vi "Aula03_25022026_Medidor.vi"() -> (0 "Corrente fase C":dynamicdata(graph), 1 "Corrente Fase B":dynamicdata(graph), 2 "Tensão Fase B":dynamicdata(graph), 4 "Tensão Fase C":dynamicdata(graph), 5 "Corrente Fase A":dynamicdata(graph), 6 "Tensão fase A":dynamicdata(graph))   [LabVIEW 2020]
panel:
  out "Fase C":string[][](table)
  out "Fase B":string[][](table)
  out "Fase A":string[][](table)
  out "Fase A":string[][](table)
  out "Table":string[][](table)
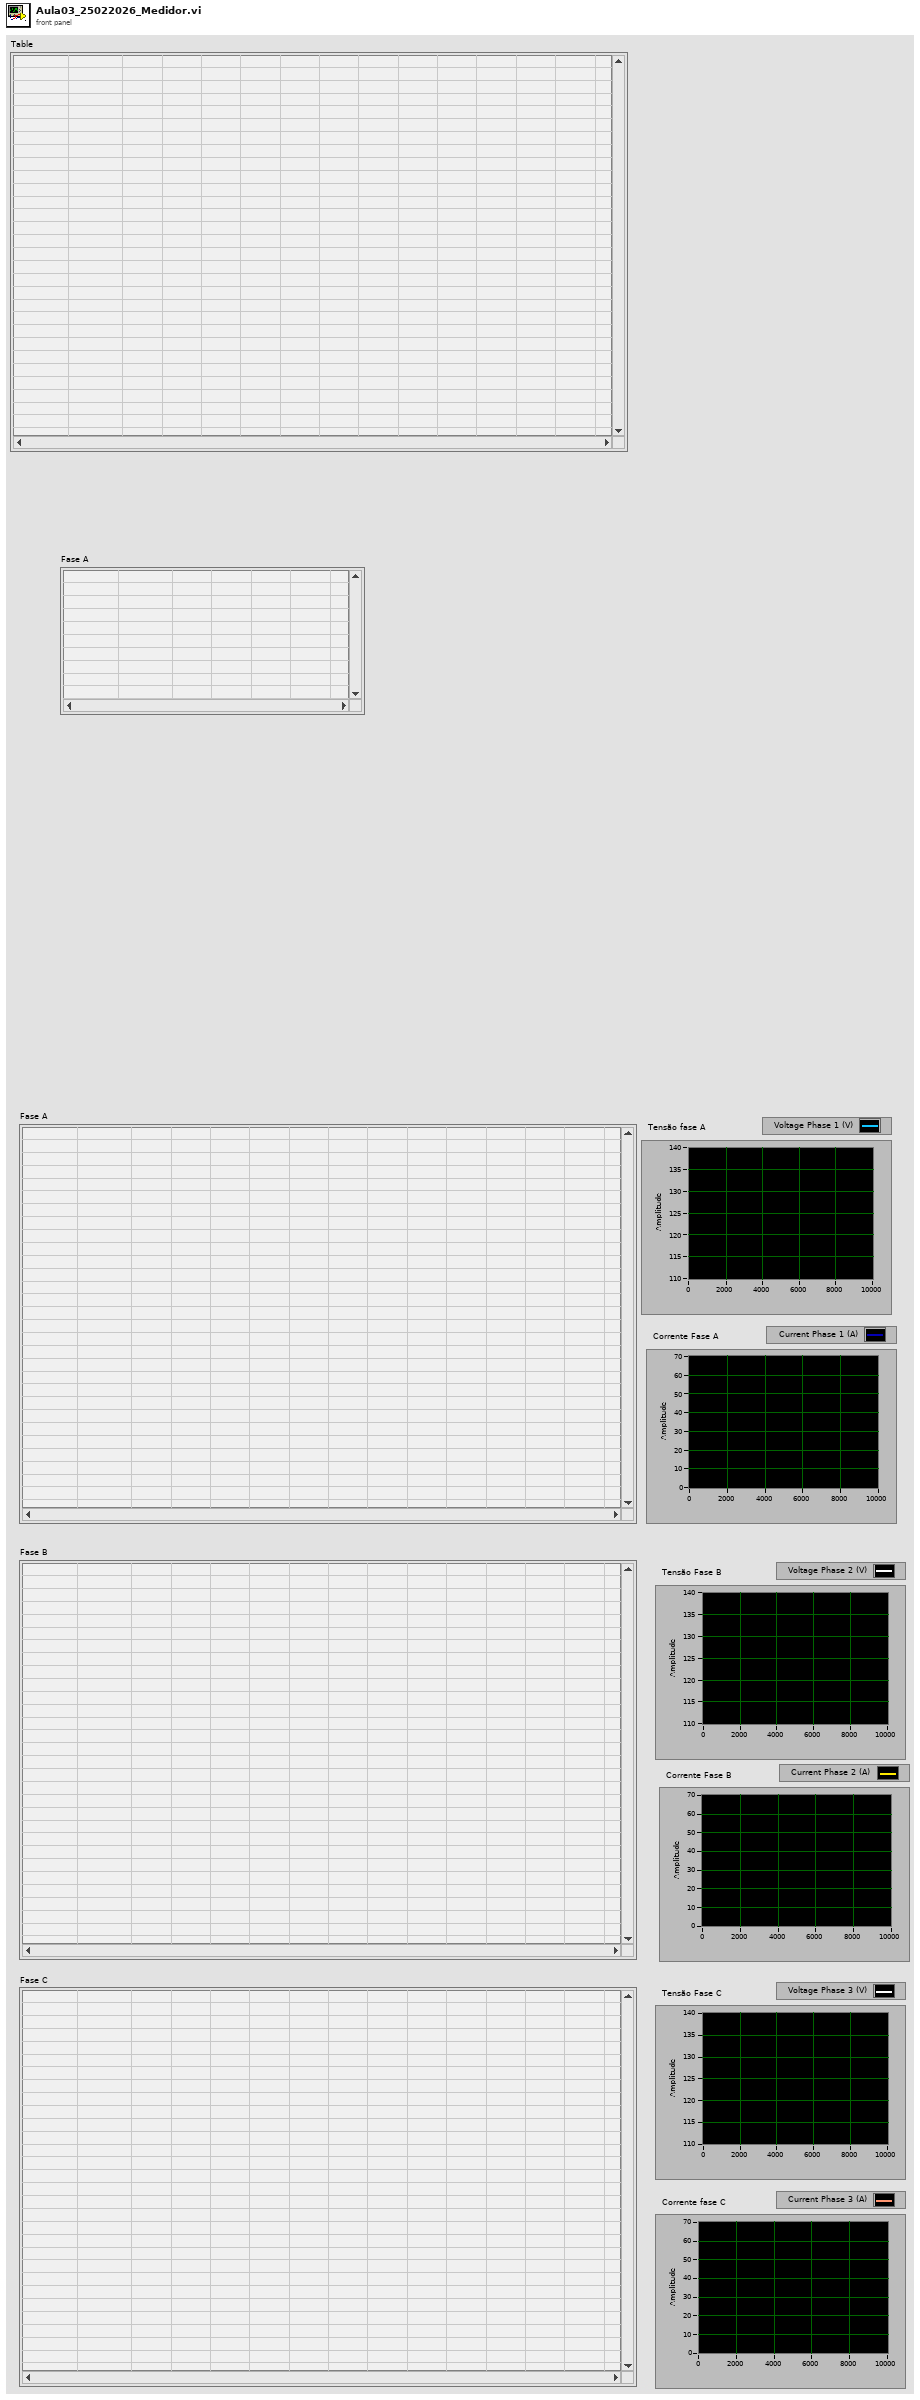
[diagram p1: front panel]
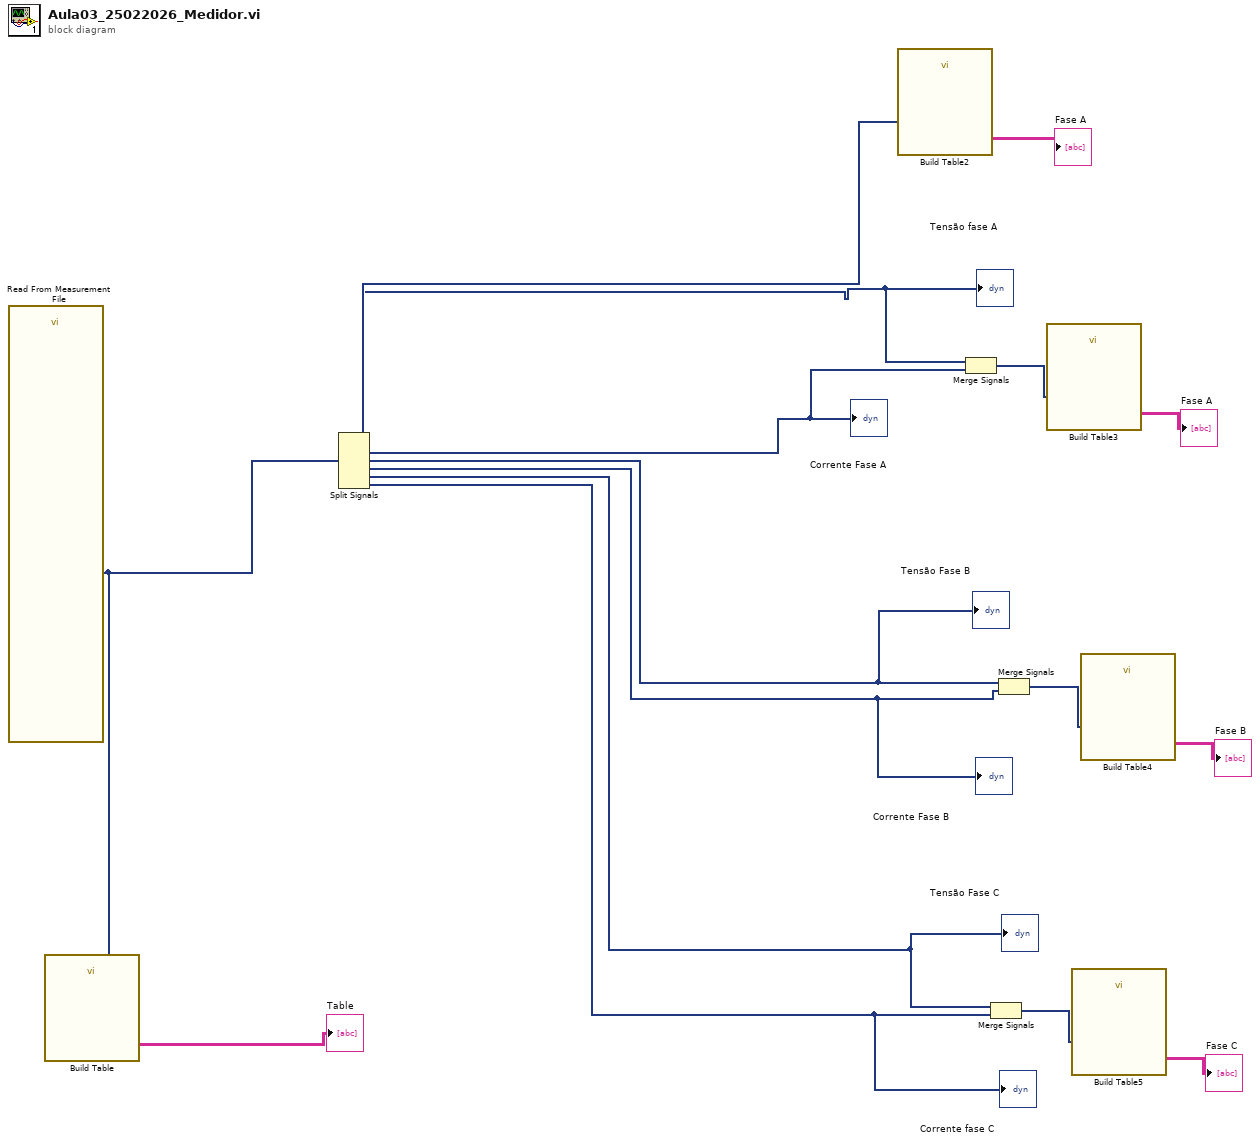
[diagram p0: block diagram]
diagram:
  n1 = call "Read From Measurement File"() -> ("Signals"=w14:dynamicdata)  [unwired: 6 in, 5 out]
  n2 = call "Build Table"("Signals"=w14) -> ("Table"=→"Table":string[][])  [unwired: 4 in, 6 out]
  n3 = Split Signals(w14) -> (w15:dynamicdata, w13:dynamicdata, w12:dynamicdata, w6:dynamicdata, w5:dynamicdata, w2:dynamicdata, w1:dynamicdata)  [unwired: 7 in]
  "Tensão fase A" <- w13
  "Corrente Fase A" <- w12
  "Tensão Fase B" <- w6
  "Corrente Fase B" <- w5
  "Tensão Fase C" <- w2
  "Corrente fase C" <- w1
  n4 = call "Build Table2"("Signals"=w15) -> ("Table"=→"Fase A":string[][])  [unwired: 4 in, 6 out]
  n5 = Merge Signals(w13, w12) -> (w11:dynamicdata)
  n6 = Merge Signals(w2, w1) -> (w4:dynamicdata)
  n7 = Merge Signals(w6, w5) -> (w9:dynamicdata)
  n8 = call "Build Table3"("Signals"=w11) -> ("Table"=→"Fase A":string[][])  [unwired: 4 in, 6 out]
  n9 = call "Build Table5"("Signals"=w4) -> ("Table"=→"Fase C":string[][])  [unwired: 4 in, 6 out]
  n10 = call "Build Table4"("Signals"=w9) -> ("Table"=→"Fase B":string[][])  [unwired: 4 in, 6 out]
